vi "Initialize Transfer.vi"(7 "component name":string, 8 "error in (no error)":errorcluster, 11 "Group Configuration":refnum<class "Group Configuration.lvclass">) -> (0 "error out":errorcluster, 3 "transfer parameters":T1[](array[typedef]))   [LabVIEW 2023, in "UDPlog.lvlib" / "UDPlog Transceiver.lvclass"]
uses:
  UDPlog Transceiver.lvclass
  Users/Public/Documents/National Instruments/NI VeriStand 2023/Custom Devices/Data Sharing Framework/Linux_x64/DSF Core.lvlibp/Classes/Configuration/Core/Group/Group Configuration.lvclass
  Typedefs/Transfer Parameters.ctl
  Configurations/Tx Transfer/UDPlog Transfer Tx Configuration.lvclass
  Configurations/Tx Transfer/UDPlog Transfer Tx Configuration.lvclass/UDPlog Transfer Tx Configuration.ctl
  Configurations/Rx Transfer/UDPlog Transfer Rx Configuration.lvclass
  Configurations/Rx Transfer/UDPlog Transfer Rx Configuration.lvclass/UDPlog Transfer Rx Configuration.ctl
  Users/Public/Documents/National Instruments/NI VeriStand 2023/Custom Devices/Data Sharing Framework/Linux_x64/DSF Core.lvlibp/Classes/Configuration/Core/Transfer/Transfer Configuration.lvclass
  C:/Users/Public/Documents/National Instruments/NI VeriStand 2023/Custom Devices/Data Sharing Framework/Linux_x64/DSF Core.lvlibp/Classes/Configuration/Core/Core Configuration.lvclass
  Users/Public/Documents/National Instruments/NI VeriStand 2023/Custom Devices/Data Sharing Framework/Linux_x64/DSF Core.lvlibp/Classes/Configuration/Core/Core Configuration.lvclass
panel:
  out "max buffer size":u64
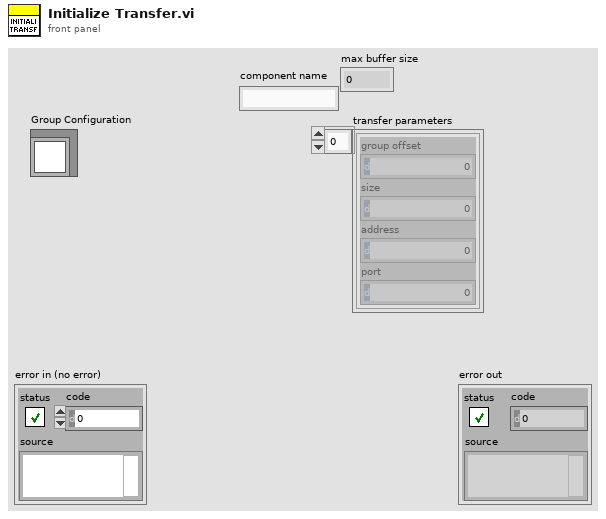
[diagram p1: front panel]
types:
  T1 = typedef "UDPlog.lvlib/UDPlog Transceiver.lvclass/Transfer Parameters.ctl" = cluster{"group offset":u64, "size":u64, "address":u32, "port":u16}
  T2 = typedef "DSF Core.lvlibp/Group Configuration.lvclass/Core Group Configuration.ctl" = cluster{"name":string, "direction":T3, "cycle timing":T4, "timeout behavior":T5, "enable conversion":bool}
  T3 = typedef "DSF Core.lvlibp/DSF Direction.ctl" = enum8{"Tx", "Rx"}
  T4 = typedef "DSF Core.lvlibp/DSF Timing Info.ctl" = cluster{"priority":u64, "decimation":u64, "offset":u64}
  T5 = typedef "DSF Core.lvlibp/DSF Timeout Behavior.ctl" = enum8{"Increment Late Count", "Throw Error"}
  T6 = typedef "DSF Core.lvlibp/DSF Settings Info.ctl" = cluster{"component":string, "values":cluster{"key":string, "value":string}[]}
  T7 = typedef "Tx Transfer Settings.ctl" = cluster{"address":u32, "port":u16}
  T8 = typedef "Rx Transfer Settings.ctl" = cluster{"address":u32, "port":u16}
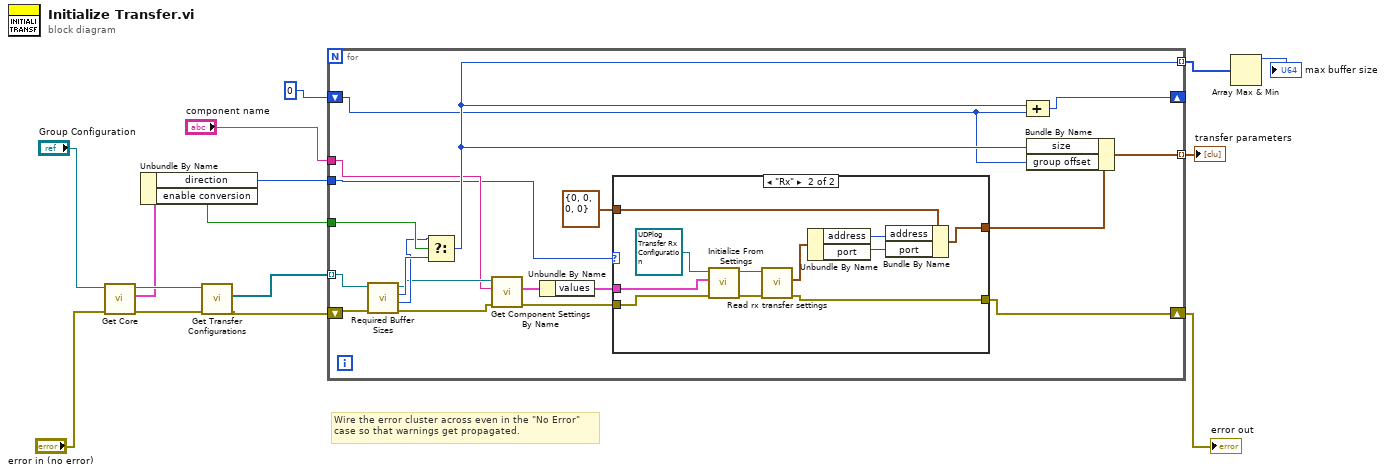
[diagram p0: block diagram]
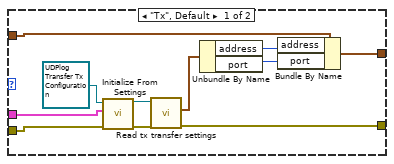
[diagram p2: hidden frame]
diagram:
  # "Wire the error cluster across even in the \"No Error\"\ncase so that warnings get propagated."
  n1 = call "Get Core.vi"("error in (no error)"="error in (no error)", "Group Configuration in"="Group Configuration") -> ("error out"=w14:errorcluster, "core"=w11:T2, "Group Configuration out"=w12:refnum<class "Group Configuration.lvclass">)  [unwired: 7 in]
  n2 = Unbundle By Name(w11) -> ("direction"=w8:T3, "enable conversion"=w7:bool)
  n3 = call "Get Transfer Configurations.vi"("error in (no error)"=w14, "Group Configuration in"=w12) -> ("error out"=w6:errorcluster, "Transfer Configurations"=w5:refnum<class "Transfer Configuration.lvclass">[])  [unwired: 7 in, 1 out]
  n4 = for {
    tunnel: "component name" -> [w25]
    shift-right: [w28] -> _
    shift-left: u64 0 -> [w16]
    tunnel: w8 -> [w23]
    tunnel: w7 -> [w32]
    tunnel: w5 -> [w34] mode=indexing
    tunnel: [w29] -> w4 mode=indexing
    tunnel: [w19] -> w2 mode=indexing
    shift-right: [w17] -> w1
    shift-left: w6 -> [w33]
    n5 = call-dynamic "Required Buffer Sizes.vi"("error in (no error)"=w33, "Transfer Configuration in"=w34) -> ("error out"=w26:errorcluster, "string size"=w30:u64, "engine size"=w31:u64, "Transfer Configuration out"=w27:refnum<class "Transfer Configuration.lvclass">)  [unwired: 6 in]
    n6 = Select(t=w30, s=w32, f=w31) -> (s? t:f=w29:u64)
    n7 = call "Get Component Settings By Name.vi"("error in (no error)"=w26, "component name"=w25, "Runtime Configuration in"=w27) -> ("error out"=w21:errorcluster, "component settings"=w22:T6)  [unwired: 6 in, 1 out]
    n8 = Unbundle By Name(w22) -> ("values"=w18:cluster{"key":string, "value":string}[])
    n9 = case shown="\"Rx\"" w23 {
      tunnel: T1 {"group offset"=0, "size"=0, "address"=0, "port"=0} ("transfer") -> [w45 w54]
      tunnel: w18 -> [w42 w51]
      tunnel: w21 -> [w41 w50]
      tunnel: [w44 w53] -> w20
      tunnel: [w37 w47] -> w17
      frame "Tx", Default {
        n10 = call-dynamic "Initialize From Settings.vi"("error in (no error)"=w41, "settings"=w42, "UDPlog Transfer Tx Configuration in"=refnum<class "UDPlog Transfer Tx Configuration.lvclass"> refnum ("UDPlog.lvlib:UDPlog Transfer Tx Configuration.lvclass")) -> ("error out"=w39:errorcluster, "UDPlog Transfer Tx Configuration out"=w40:refnum<class "UDPlog Transfer Tx Configuration.lvclass">)  [unwired: 7 in]
        n11 = call "Read tx transfer settings.vi"("error in (no error)"=w39, "UDPlog Transfer Tx Configuration in"=w40) -> ("error out"=w37:errorcluster, "tx transfer settings"=w38:T7)  [unwired: 7 in, 1 out]
        n12 = Unbundle By Name(w38) -> ("address"=w36:u32, "port"=w35:u16)
        n13 = Bundle By Name(cluster=w45, "address"=w36, "port"=w35) -> (w44:T1)
      }
      frame "Rx" {
        n14 = call-dynamic "Initialize From Settings.vi"("error in (no error)"=w50, "settings"=w51, "UDPlog Transfer Rx Configuration in"=refnum<class "UDPlog Transfer Rx Configuration.lvclass"> refnum ("UDPlog.lvlib:UDPlog Transfer Rx Configuration.lvclass")) -> ("error out"=w48:errorcluster, "UDPlog Transfer Rx Configuration out"=w49:refnum<class "UDPlog Transfer Rx Configuration.lvclass">)  [unwired: 7 in]
        n15 = call "Read rx transfer settings.vi"("error in (no error)"=w48, "UDPlog Transfer Rx Configuration in"=w49) -> ("error out"=w47:errorcluster, "rx transfer settings"=w46:T8)  [unwired: 7 in, 1 out]
        n16 = Unbundle By Name(w46) -> ("address"=w56:u32, "port"=w55:u16)
        n17 = Bundle By Name(cluster=w54, "address"=w56, "port"=w55) -> (w53:T1)
      }
    }
    n18 = Compound Arithmetic op=ADD(w29, w16) -> (w28:u64)
    n19 = Bundle By Name(cluster=w20, "size"=w29, "group offset"=w16) -> (w19:T1)
  }
  "error out" <- w1
  "transfer parameters" <- w2
  n20 = Array Max & Min(array=w4) -> (max value=→"max buffer size":u64)  [unwired: 3 out]
